vi "PRIME Detector wait for Request Complete message.vi"(8 "error in":errorcluster, 11 "connection ID":refnum<k5>) -> (0 "error out":errorcluster, 3 "response":string)   [LabVIEW 2021, in "PRIME Detector.lvclass"]
uses:
  PRIME Detector.lvclass
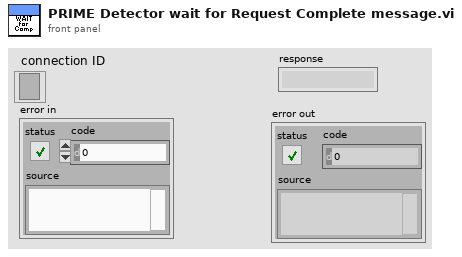
[diagram p1: front panel]
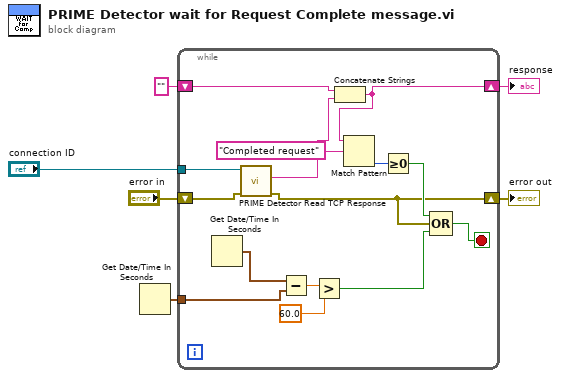
[diagram p0: block diagram]
diagram:
  n1 = Get Date/Time In Seconds() -> (seconds since 1Jan1904=w1:timestamp)
  n2 = while {
    tunnel: "connection ID" -> [w21]
    shift-right: [w16] -> w4
    shift-left: "error in" -> [w20]
    shift-right: [w13] -> w2
    shift-left: "" -> [w12]
    tunnel: w1 -> [w10]
    stop <- w15 stop-if-true
    n3 = Get Date/Time In Seconds() -> (seconds since 1Jan1904=w11:timestamp)
    n4 = call "PRIME Detector Read TCP Response.vi"("error in (no error)"=w20, "connection ID"=w21) -> ("error out"=w16:errorcluster, "response message"=w14:string)  [unwired: 6 in, 2 out]
    n5 = Subtract(x=w11, y=w10) -> (x-y=w9:dbl)
    n6 = Greater?(x=w9, y=60.0) -> (0:w7:bool)
    n7 = Concatenate Strings(w12, w14) -> (w13:string)
    n8 = Match Pattern(string=w13, regular expression="Completed request") -> (offset past match=w18:i32)  [unwired: 1 in, 3 out]
    n9 = Greater Or Equal To 0?(x=w18) -> (x >= 0?=w17:bool)
    n10 = Compound Arithmetic op=OR(w17, w16, w7) -> (w15:bool)
  }
  "error out" <- w4
  "response" <- w2
